vi "Hardware - NI 9220-1 (AI) Host.vi"() -> ()   [LabVIEW 2015, in "ECS-Host.lvlib"]
uses:
  ECS-Host.lvlib
panel:
  out "Analog":sgl[](array[numeric]) caption="[V]"
  out "FPGAReadError":bool
  # "CH0\nCH1\nCH2\nCH3\nCH4\nCH5\nCH6\nCH7\nCH8\nCH9\nCH10\nCH11\nCH12\nCH13\nCH14\nCH15"
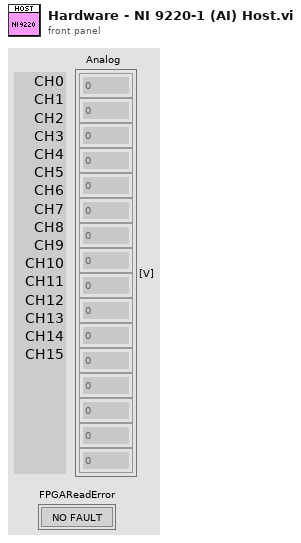
[diagram p1: front panel]
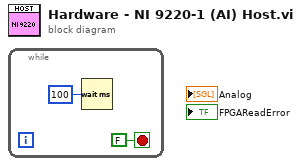
[diagram p0: block diagram]
diagram:
  n1 = while {
    stop <- FALSE stop-if-true
    n2 = Wait (ms)(milliseconds to wait=u32 100) -> ()  [unwired: 1 out]
  }
